vi "sample2(BasicRW).vi"() -> ()   [LabVIEW 2011]
panel:
  out "PRESENT POSITION":u16
  in  "ID":u8=1 max=253
  in  "Baudrate":u32=1000000
  in  "COM":refnum<visa-resource-name> caption="COMポート"
  in  "STOP":bool
  in  "GOAL POSITION":u16(knob) scale=0.0..4095.0
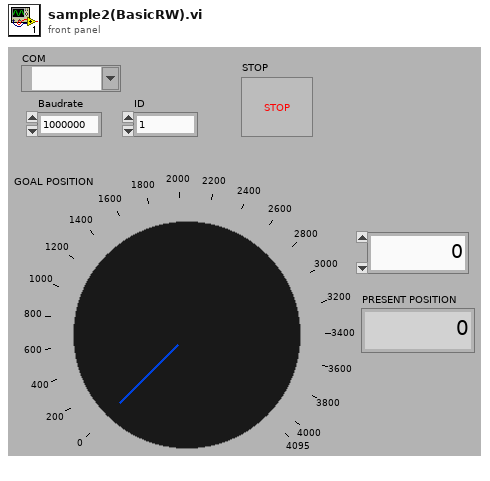
[diagram p1: front panel]
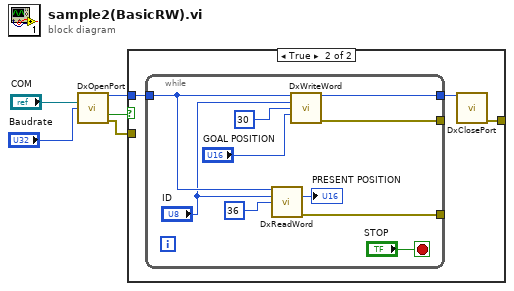
[diagram p0: block diagram]
diagram:
  n1 = call "DxOpenPort.vi"("port"="COM", "baudrate"="Baudrate") -> ("dvid"=w3:u32, "成功"=w2:bool, "エラー出力"=w1:errorcluster)  [unwired: 11 in]
  n2 = case shown="TRUE" w2 {
    tunnel: w3 -> [_ w8]
    tunnel: w1 -> [_ _]
    tunnel: [_ w6] -> _
    frame False {
    }
    frame True {
      n3 = while {
        tunnel: w8 -> [w14]
        tunnel: [w15] -> w7
        tunnel: [w12] -> _
        tunnel: [w11] -> _
        stop <- "STOP" stop-if-true
        n4 = call "DxReadWord.vi"("dvid in"=w14, "id"="ID", "address"=u16 36) -> ("data out"=→"PRESENT POSITION":u16, "エラー出力"=w11:errorcluster)  [unwired: 9 in, 2 out]
        n5 = call "DxWriteWord.vi"("dvid in"=w14, "id"="ID", "address"=u16 30, "data in"="GOAL POSITION") -> ("dvid out"=w15:u32, "エラー出力"=w12:errorcluster)  [unwired: 9 in, 1 out]
      }
      n6 = call "DxClosePort.vi"("dvid"=w7) -> ("エラー出力"=w6:errorcluster)  [unwired: 13 in, 1 out]
    }
  }
